vi "Control CP Voltage.vi"(8 "error out":errorcluster, 11 "CP to HD/Cycle":i32(ring)=1 items=["CP HDC 35V", "CP HDC 40.25V", "CP HDC 27.5V", "CP HDC 30.5V", "CP HDC 44V"]) -> (0 "error out 2":errorcluster, 2 "V_Out":string, 3 "Cmd Out":string)   [LabVIEW 2012]
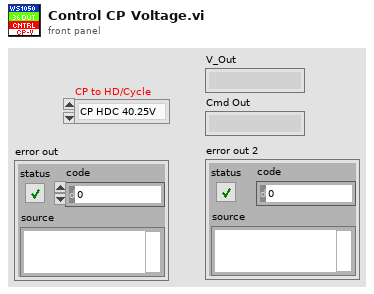
[diagram p1: front panel]
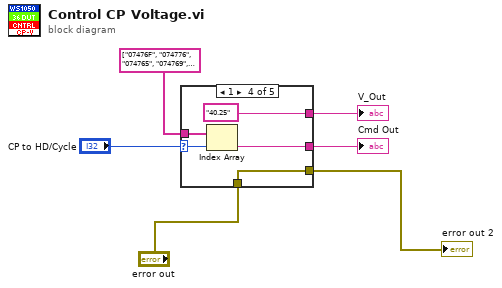
[diagram p0: block diagram]
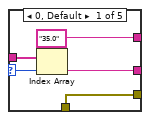
[diagram p2: hidden frame]
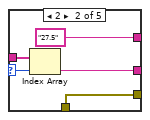
[diagram p3: hidden frame]
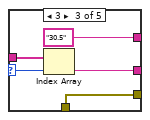
[diagram p4: hidden frame]
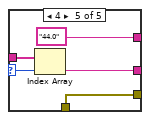
[diagram p5: hidden frame]
diagram:
  n1 = case shown="1" "CP to HD/Cycle" {
    selector: "CP to HD/Cycle" -> [w10 w15 w20 w24 w29]
    tunnel: string[] ["07476F", "074776", "074765", "074769", "07477B"] -> [w11 w16 w21 w26 w31]
    tunnel: [w9 w14 w19 w25 w30] -> w1
    tunnel: ["35.0" ("Data Out") "27.5" ("Data Out") "30.5" ("Data Out") "40.25" ("Data Out") "44.0" ("Data Out")] -> w2
    tunnel: [w7 w12 w17 w22 w27] -> w3
    tunnel: "error out" -> [w7 w12 w17 w22 w27]
    frame 0, Default {
      n2 = Index Array(array=w11, index=w10) -> (element=w9:string)
    }
    frame 2 {
      n3 = Index Array(array=w16, index=w15) -> (element=w14:string)
    }
    frame 3 {
      n4 = Index Array(array=w21, index=w20) -> (element=w19:string)
    }
    frame 1 {
      n5 = Index Array(array=w26, index=w24) -> (element=w25:string)
    }
    frame 4 {
      n6 = Index Array(array=w31, index=w29) -> (element=w30:string)
    }
  }
  "error out 2" <- w3
  "V_Out" <- w2
  "Cmd Out" <- w1
